vi "Last Dance.vi"() -> ()   [LabVIEW 2014]
doc: "Last Dance\n\nOnce inside the ring, it actively executes defensive commands based off of Determine State.vi\nIf Determine State.vi returns:\n\nSpin Move, then it will run the Spin Move.vi\nRight Bumped, then it will reverse left and then move forward\nLeft Bumped, then it will reverse right and then move forward\nFront Bumped, then push forward\n\nOut of Bounds, then it will reverse\nOut of Bounds and Right Bumped, then it will reverse left and then move right\nOut of Bounds and Left Bumped, then it will reverse right and then move left\nOut of Bounds and Front Bumped, theni t will push forward\n\nBeverly Abadines\nPHY 350\nBAP7s"
uses:
  <vilib>/NXT/Block Support/NXT_InputPort.ctl
  <vilib>/NXT/NXTIO Xnodes/NXTIONodeSubVIs/NXTMotorSteeringOn.vi
  <vilib>/NXT/NXTIO Xnodes/NXTIOXNode/NXTIO.xnode
  <vilib>/NXT/Block Support/NXT_OutputPort.ctl
  <vilib>/NXT/Subs/LVHSConnector.ctl
  <vilib>/NXT/LegoClasses/BrickReference/BrickReference.lvclass
panel:
  in  "Front Bumper":T1=1 items=["Port 1", "Port 2", "Port 3", "Port 4"]
  # "Last Dance"
  # "Beverly Abadines\nPhys 350\nP7"
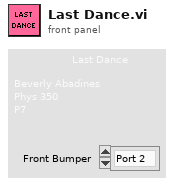
[diagram p1: front panel]
types:
  T1 = typedef "NXT_InputPort.ctl" = u32
  T2 = typedef "LVHSConnector.ctl" = refnum<class "BrickReference.lvclass">
  T3 = typedef "NXT_OutputPort.ctl" = u8
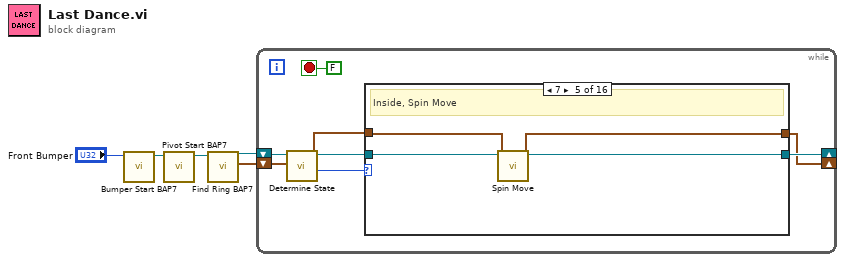
[diagram p0: block diagram]
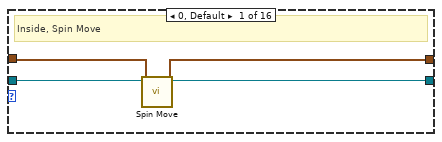
[diagram p2: hidden frame]
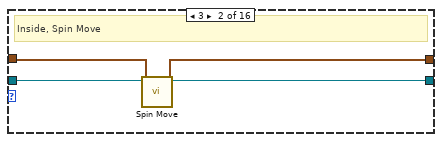
[diagram p3: hidden frame]
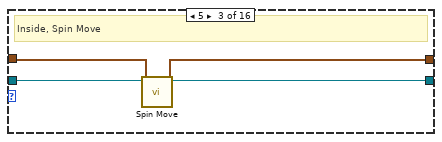
[diagram p4: hidden frame]
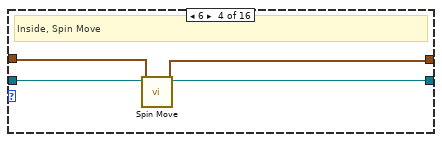
[diagram p5: hidden frame]
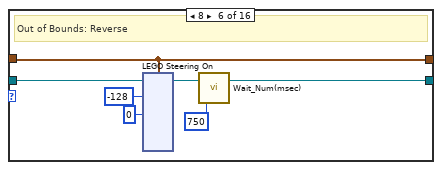
[diagram p6: hidden frame]
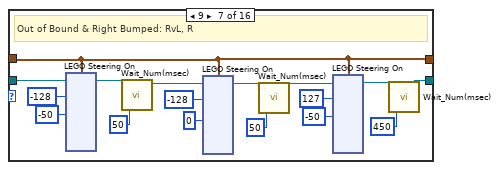
[diagram p7: hidden frame]
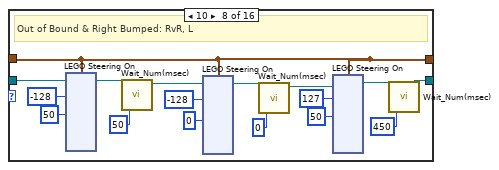
[diagram p8: hidden frame]
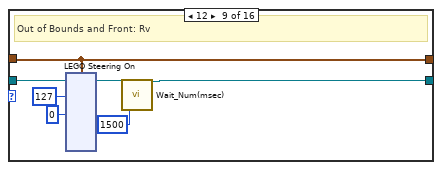
[diagram p9: hidden frame]
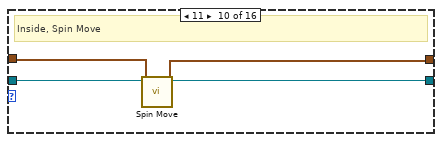
[diagram p10: hidden frame]
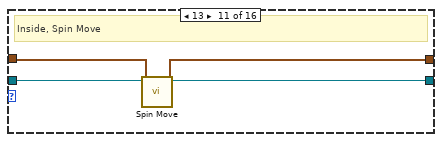
[diagram p11: hidden frame]
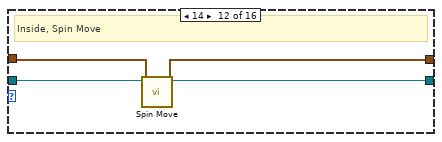
[diagram p12: hidden frame]
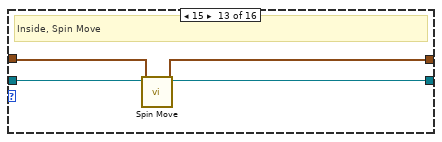
[diagram p13: hidden frame]
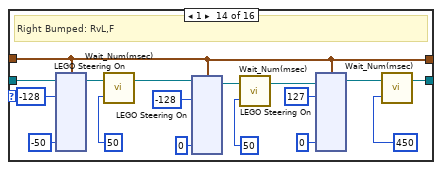
[diagram p14: hidden frame]
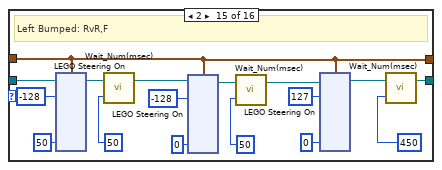
[diagram p15: hidden frame]
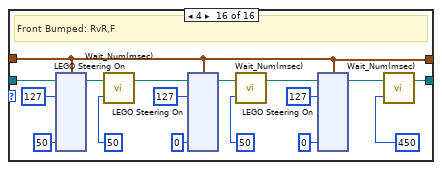
[diagram p16: hidden frame]
diagram:
  n1 = call "Bumper Start BAP7.vi"("Port (Port 1)"="Front Bumper") -> ("BrickReference out"=w3:T2)  [unwired: 10 in]
  n2 = call "Pivot Start BAP7.vi"("BrickReference in"=w3) -> ("BrickReference out"=w5:T2)  [unwired: 10 in]
  n3 = call "Find Ring BAP7.vi"("BrickReference in"=w5) -> ("Motor Out"=w1:cluster{"Port":T3, "Port":T3}, "BrickReference Out"=w2:T2)  [unwired: 9 in]
  n4 = while {
    shift-right: [w13] -> _
    shift-left: w2 -> [w10]
    shift-right: [w12] -> _
    shift-left: w1 -> [w8]
    stop <- FALSE stop-if-true
    n5 = call "Determine State.vi"("Motor In"=w8, "Ref in"=w10) -> ("State"=w9:i16, "Motor Out"=w7:cluster{"Port":T3, "Port":T3}, "Ref Out"=w6:T2)  [unwired: 7 in]
    n6 = case shown="7" w9 {
      tunnel: [w17 w21 w25 w29 w33 w35 w56 w97 w131 w149 w153 w157 w161 w175 w216 w257] -> w13
      tunnel: [w16 w20 w24 w28 w32 w39 w51 w92 w132 w148 w152 w156 w160 w163 w203 w245] -> w12
      tunnel: w7 -> [w15 w19 w23 w27 w31 w39 w51 w92 w132 w147 w151 w155 w159 w163 w203 w245]
      tunnel: w6 -> [w14 w18 w22 w26 w30 w40 w65 w106 w137 w146 w150 w154 w158 w174 w215 w256]
      frame 0, Default {
        # "Inside, Spin Move"
        n7 = call "Spin Move.vi"("Motor In"=w15, "Ref In"=w14) -> ("Motor Out"=w16:cluster{"Port":T3, "Port":T3}, "Ref Out"=w17:T2)  [unwired: 8 in]
      }
      frame 3 {
        # "Inside, Spin Move"
        n8 = call "Spin Move.vi"("Motor In"=w19, "Ref In"=w18) -> ("Motor Out"=w20:cluster{"Port":T3, "Port":T3}, "Ref Out"=w21:T2)  [unwired: 8 in]
      }
      frame 5 {
        # "Inside, Spin Move"
        n9 = call "Spin Move.vi"("Motor In"=w23, "Ref In"=w22) -> ("Motor Out"=w24:cluster{"Port":T3, "Port":T3}, "Ref Out"=w25:T2)  [unwired: 8 in]
      }
      frame 6 {
        # "Inside, Spin Move"
        n10 = call "Spin Move.vi"("Motor In"=w27, "Ref In"=w26) -> ("Motor Out"=w28:cluster{"Port":T3, "Port":T3}, "Ref Out"=w29:T2)  [unwired: 8 in]
      }
      frame 7 {
        # "Inside, Spin Move"
        n11 = call "Spin Move.vi"("Motor In"=w31, "Ref In"=w30) -> ("Motor Out"=w32:cluster{"Port":T3, "Port":T3}, "Ref Out"=w33:T2)  [unwired: 8 in]
      }
      frame 8 {
        # "Out of Bounds: Reverse"
        n12 = xnode "LEGO Steering On"("Steering 1"=0, "Power 1"=-128, "Motors"=w39, "NXT/EV3"=w40) -> ("NXT/EV3"=w36:T2)
        n13 = call <vilib>:"Wait_Num(msec).vi"("Time (100 msec)"=u32 750, "NXT/EV3"=w36) -> ("NXT/EV3"=w35:T2)  [unwired: 2 in]
      }
      frame 9 {
        # "Out of Bound & Right Bumped: RvL, R"
        n14 = xnode "LEGO Steering On"("Steering 1"=-50, "Power 1"=-128, "Motors"=w51, "NXT/EV3"=w65) -> ("NXT/EV3"=w62:T2)
        n15 = call <vilib>:"Wait_Num(msec).vi"("Time (100 msec)"=u32 50, "NXT/EV3"=w62) -> ("NXT/EV3"=w50:T2)  [unwired: 2 in]
        n16 = xnode "LEGO Steering On"("Steering 1"=0, "Power 1"=-128, "Motors"=w51, "NXT/EV3"=w50) -> ("NXT/EV3"=w54:T2)
        n17 = call <vilib>:"Wait_Num(msec).vi"("Time (100 msec)"=u32 50, "NXT/EV3"=w54) -> ("NXT/EV3"=w49:T2)  [unwired: 2 in]
        n18 = xnode "LEGO Steering On"("Steering 1"=-50, "Power 1"=127, "Motors"=w51, "NXT/EV3"=w49) -> ("NXT/EV3"=w59:T2)
        n19 = call <vilib>:"Wait_Num(msec).vi"("Time (100 msec)"=u32 450, "NXT/EV3"=w59) -> ("NXT/EV3"=w56:T2)  [unwired: 2 in]
      }
      frame 10 {
        # "Out of Bound & Right Bumped: RvR, L"
        n20 = xnode "LEGO Steering On"("Steering 1"=50, "Power 1"=-128, "Motors"=w92, "NXT/EV3"=w106) -> ("NXT/EV3"=w103:T2)
        n21 = call <vilib>:"Wait_Num(msec).vi"("Time (100 msec)"=u32 50, "NXT/EV3"=w103) -> ("NXT/EV3"=w91:T2)  [unwired: 2 in]
        n22 = xnode "LEGO Steering On"("Steering 1"=0, "Power 1"=-128, "Motors"=w92, "NXT/EV3"=w91) -> ("NXT/EV3"=w95:T2)
        n23 = call <vilib>:"Wait_Num(msec).vi"("Time (100 msec)"=u32 0, "NXT/EV3"=w95) -> ("NXT/EV3"=w90:T2)  [unwired: 2 in]
        n24 = xnode "LEGO Steering On"("Steering 1"=50, "Power 1"=127, "Motors"=w92, "NXT/EV3"=w90) -> ("NXT/EV3"=w100:T2)
        n25 = call <vilib>:"Wait_Num(msec).vi"("Time (100 msec)"=u32 450, "NXT/EV3"=w100) -> ("NXT/EV3"=w97:T2)  [unwired: 2 in]
      }
      frame 12 {
        # "Out of Bounds and Front: Rv"
        n26 = xnode "LEGO Steering On"("Steering 1"=0, "Power 1"=127, "Motors"=w132, "NXT/EV3"=w137) -> ("NXT/EV3"=w134:T2)
        n27 = call <vilib>:"Wait_Num(msec).vi"("Time (100 msec)"=u32 1500, "NXT/EV3"=w134) -> ("NXT/EV3"=w131:T2)  [unwired: 2 in]
      }
      frame 11 {
        # "Inside, Spin Move"
        n28 = call "Spin Move.vi"("Motor In"=w147, "Ref In"=w146) -> ("Motor Out"=w148:cluster{"Port":T3, "Port":T3}, "Ref Out"=w149:T2)  [unwired: 8 in]
      }
      frame 13 {
        # "Inside, Spin Move"
        n29 = call "Spin Move.vi"("Motor In"=w151, "Ref In"=w150) -> ("Motor Out"=w152:cluster{"Port":T3, "Port":T3}, "Ref Out"=w153:T2)  [unwired: 8 in]
      }
      frame 14 {
        # "Inside, Spin Move"
        n30 = call "Spin Move.vi"("Motor In"=w155, "Ref In"=w154) -> ("Motor Out"=w156:cluster{"Port":T3, "Port":T3}, "Ref Out"=w157:T2)  [unwired: 8 in]
      }
      frame 15 {
        # "Inside, Spin Move"
        n31 = call "Spin Move.vi"("Motor In"=w159, "Ref In"=w158) -> ("Motor Out"=w160:cluster{"Port":T3, "Port":T3}, "Ref Out"=w161:T2)  [unwired: 8 in]
      }
      frame 1 {
        # "Right Bumped: RvL,F"
        n32 = xnode "LEGO Steering On"("Steering 1"=-50, "Power 1"=-128, "Motors"=w163, "NXT/EV3"=w174) -> ("NXT/EV3"=w171:T2)
        n33 = call <vilib>:"Wait_Num(msec).vi"("Time (100 msec)"=u32 50, "NXT/EV3"=w171) -> ("NXT/EV3"=w164:T2)  [unwired: 2 in]
        n34 = xnode "LEGO Steering On"("Steering 1"=0, "Power 1"=-128, "Motors"=w163, "NXT/EV3"=w164) -> ("NXT/EV3"=w168:T2)
        n35 = call <vilib>:"Wait_Num(msec).vi"("Time (100 msec)"=u32 50, "NXT/EV3"=w168) -> ("NXT/EV3"=w162:T2)  [unwired: 2 in]
        n36 = xnode "LEGO Steering On"("Steering 1"=0, "Power 1"=127, "Motors"=w163, "NXT/EV3"=w162) -> ("NXT/EV3"=w169:T2)
        n37 = call <vilib>:"Wait_Num(msec).vi"("Time (100 msec)"=u32 450, "NXT/EV3"=w169) -> ("NXT/EV3"=w175:T2)  [unwired: 2 in]
      }
      frame 2 {
        # "Left Bumped: RvR,F"
        n38 = xnode "LEGO Steering On"("Steering 1"=50, "Power 1"=-128, "Motors"=w203, "NXT/EV3"=w215) -> ("NXT/EV3"=w212:T2)
        n39 = call <vilib>:"Wait_Num(msec).vi"("Time (100 msec)"=u32 50, "NXT/EV3"=w212) -> ("NXT/EV3"=w205:T2)  [unwired: 2 in]
        n40 = xnode "LEGO Steering On"("Steering 1"=0, "Power 1"=-128, "Motors"=w203, "NXT/EV3"=w205) -> ("NXT/EV3"=w209:T2)
        n41 = call <vilib>:"Wait_Num(msec).vi"("Time (100 msec)"=u32 50, "NXT/EV3"=w209) -> ("NXT/EV3"=w204:T2)  [unwired: 2 in]
        n42 = xnode "LEGO Steering On"("Steering 1"=0, "Power 1"=127, "Motors"=w203, "NXT/EV3"=w204) -> ("NXT/EV3"=w210:T2)
        n43 = call <vilib>:"Wait_Num(msec).vi"("Time (100 msec)"=u32 450, "NXT/EV3"=w210) -> ("NXT/EV3"=w216:T2)  [unwired: 2 in]
      }
      frame 4 {
        # "Front Bumped: RvR,F"
        n44 = xnode "LEGO Steering On"("Steering 1"=50, "Power 1"=127, "Motors"=w245, "NXT/EV3"=w256) -> ("NXT/EV3"=w253:T2)
        n45 = call <vilib>:"Wait_Num(msec).vi"("Time (100 msec)"=u32 50, "NXT/EV3"=w253) -> ("NXT/EV3"=w246:T2)  [unwired: 2 in]
        n46 = xnode "LEGO Steering On"("Steering 1"=0, "Power 1"=127, "Motors"=w245, "NXT/EV3"=w246) -> ("NXT/EV3"=w250:T2)
        n47 = call <vilib>:"Wait_Num(msec).vi"("Time (100 msec)"=u32 50, "NXT/EV3"=w250) -> ("NXT/EV3"=w244:T2)  [unwired: 2 in]
        n48 = xnode "LEGO Steering On"("Steering 1"=0, "Power 1"=127, "Motors"=w245, "NXT/EV3"=w244) -> ("NXT/EV3"=w251:T2)
        n49 = call <vilib>:"Wait_Num(msec).vi"("Time (100 msec)"=u32 450, "NXT/EV3"=w251) -> ("NXT/EV3"=w257:T2)  [unwired: 2 in]
      }
    }
  }
